vi "Int16Array Create.vi"(8 "error in (no error)":errorcluster, 11 "I16 array in":i16[](array[numeric])) -> (0 "error out":errorcluster, 3 "Int16Array DVR out":refnum<data-value>)   [LabVIEW 2015, in "MDSplus.lvlib"]
uses:
  <vilib>/MDSplus/Library/MDSplus.lvlib
  <vilib>/MDSplus/Classes/Data_Class/Array_Class/Int16Array_Class/Int16Array.lvclass
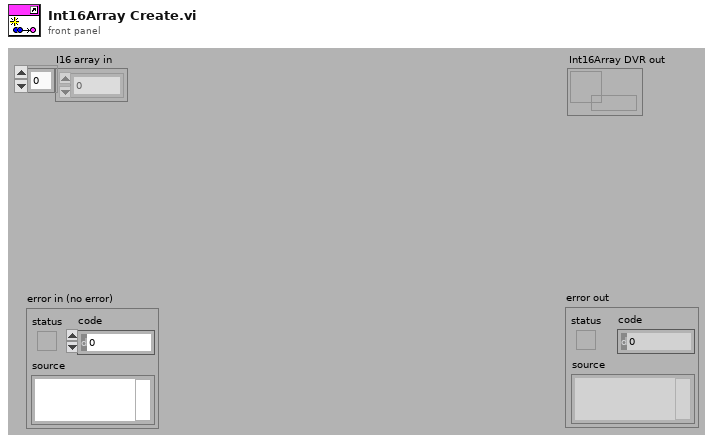
[diagram p1: front panel]
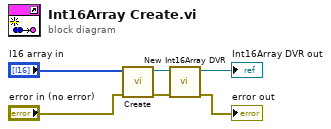
[diagram p0: block diagram]
diagram:
  n1 = call <vilib>:"Create.vi"("error in (no error)"="error in (no error)", "I16 array in"="I16 array in") -> ("error out"=w3:errorcluster, "Int16Array out"=w4:refnum<class "Int16Array.lvclass">)  [unwired: 8 in]
  n2 = call <vilib>:"New Int16Array DVR.vi"("error in (no error)"=w3, "Int16Array in"=w4) -> ("error out"=→"error out":errorcluster, "Int16Array DVR out"=→"Int16Array DVR out":refnum<data-value>)  [unwired: 8 in]
